vi "2-6-1.vi"() -> ()   [LabVIEW 2022 SP3]
uses:
  2-6-3.vi
panel:
  in  "旋钮":dbl(knob) scale=0.0..10.0
  in  "布尔":bool
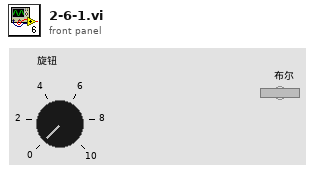
[diagram p1: front panel]
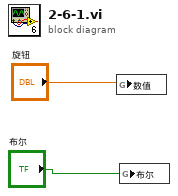
[diagram p0: block diagram]
diagram:
  n1 = global write "2-6-3.vi" "数值"("旋钮") -> ()
  n2 = global write "2-6-3.vi" "布尔"("布尔") -> ()
